vi "FGV_compteur.vi"(1 "Commande":T1) -> (0 "Read Data":u8)   [LabVIEW 2020]
uses:
  Ctrl/Ctrl_state_FGV.ctl
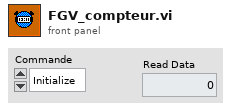
[diagram p1: front panel]
types:
  T1 = typedef "Ctrl_state_FGV.ctl" = enum16{"Initialize", "Write", "Read"}
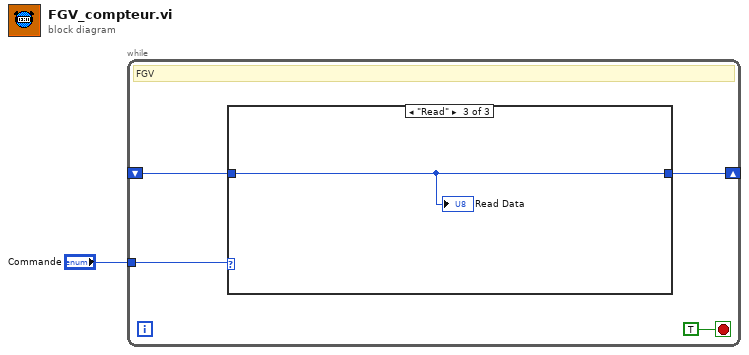
[diagram p0: block diagram]
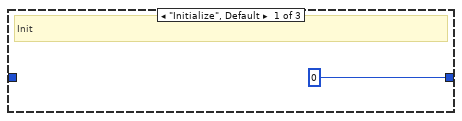
[diagram p2: hidden frame]
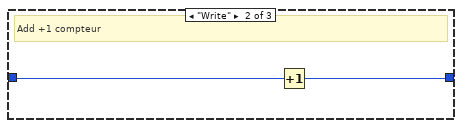
[diagram p3: hidden frame]
diagram:
  n1 = while {
    shift-right: [w3] -> _
    shift-left: _ -> [w2]
    tunnel: "Commande" -> [w4]
    stop <- TRUE stop-if-true
    # "FGV"
    n2 = case shown="\"Read\"" w4 {
      tunnel: [u8 0 w8 w9] -> w3
      tunnel: w2 -> [_ w7 w9]
      frame "Initialize", Default {
        # "Init"
      }
      frame "Write" {
        # "Add +1 compteur"
        n3 = Increment(x=w7) -> (x+1=w8:u8)
      }
      frame "Read" {
        "Read Data" <- w9
      }
    }
  }
